vi "Delete Files.vi"(8 "error in (no error)":errorcluster, 11 "Server Fixture in":refnum<class "Server Fixture.lvclass">) -> (0 "error out":errorcluster, 3 "Server Fixture out":refnum<class "Server Fixture.lvclass">)   [LabVIEW 2013, in "libssh2_integration_tests.lvlib" / "Server Fixture.lvclass"]
uses:
  Server Fixture.lvclass
  Server Fixture.lvclass/Server Fixture.ctl
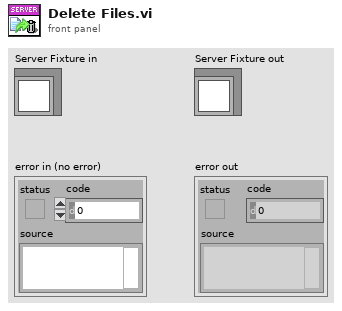
[diagram p1: front panel]
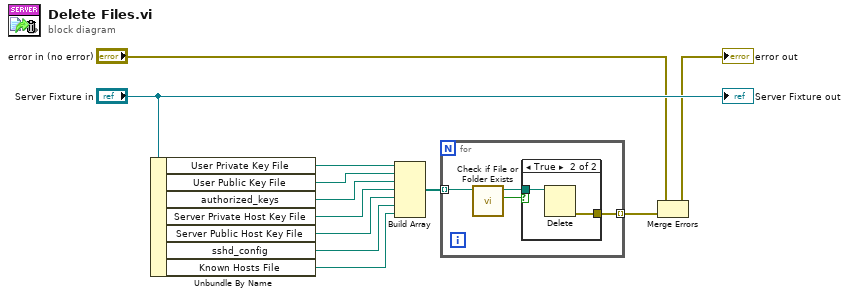
[diagram p0: block diagram]
diagram:
  n1 = Unbundle By Name("Server Fixture in") -> ("User Private Key File"=w12:path, "User Public Key File"=w10:path, "authorized_keys"=w11:path, "Server Private Host Key File"=w8:path, "Server Public Host Key File"=w6:path, "sshd_config"=w7:path, "Known Hosts File"=w1:path)
  n2 = Build Array(w12, w10, w11, w8, w6, w7, w1) -> (w9:path[])
  n3 = for {
    tunnel: [w16] -> w4 mode=indexing
    tunnel: w9 -> [w15] mode=indexing
    n4 = call <vilib>:"Check if File or Folder Exists.vi"("path"=w15) -> ("file or folder exists?"=w13:bool, "dup path"=w14:path)  [unwired: 8 in, 1 out]
    n5 = case shown="True" w13 {
      tunnel: [_ w18] -> w16
      tunnel: w14 -> [_ w17]
      frame False {
      }
      frame True {
        n6 = Delete(path (use dialog)=w17) -> (error out=w18:errorcluster)  [unwired: 4 in, 2 out]
      }
    }
  }
  n7 = Merge Errors("error in (no error)", w4) -> (→"error out":errorcluster)
  "Server Fixture out" <- "Server Fixture in"
